vi "MyTestVI.vi"() -> ()   [LabVIEW 2018]
panel:
  in  "Stop Button":bool
  in  "test":bool
  out "error out":errorcluster
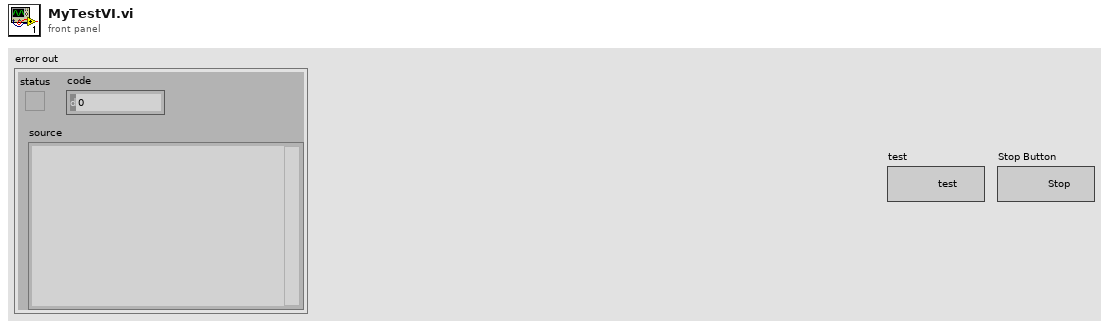
[diagram p1: front panel]
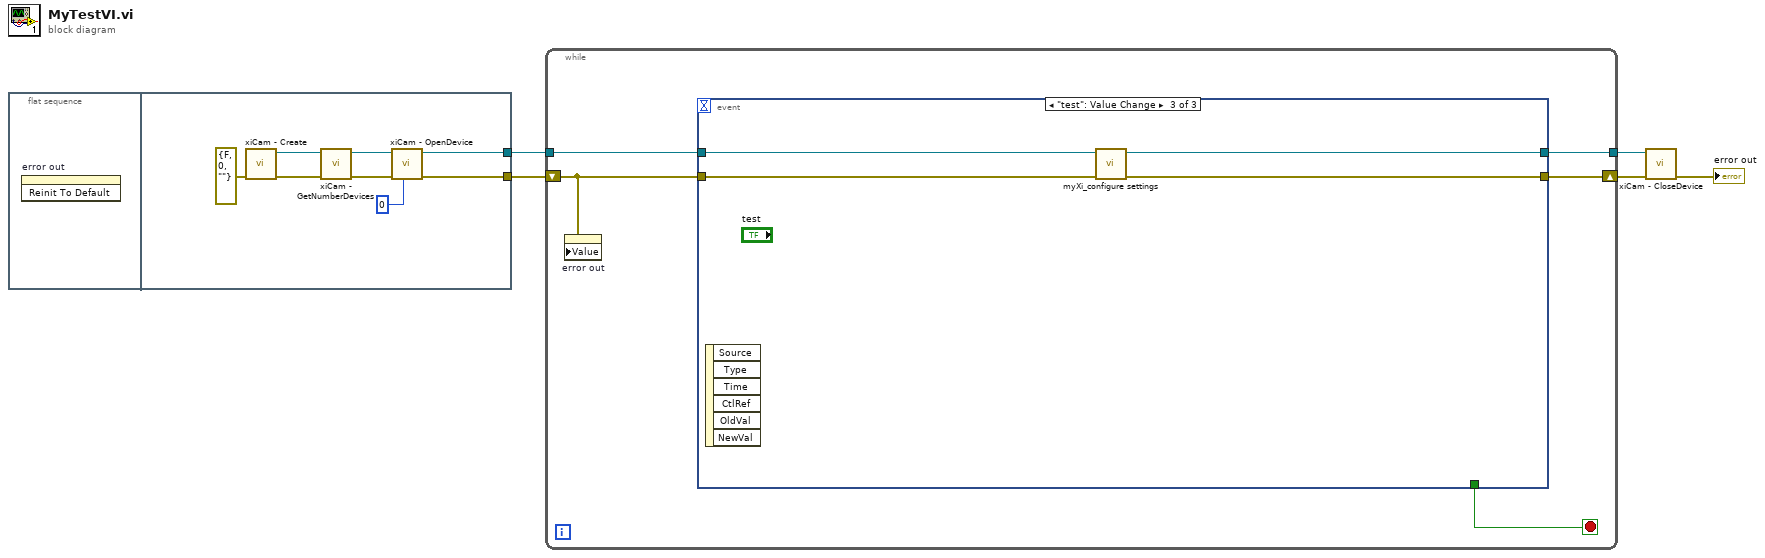
[diagram p0: block diagram]
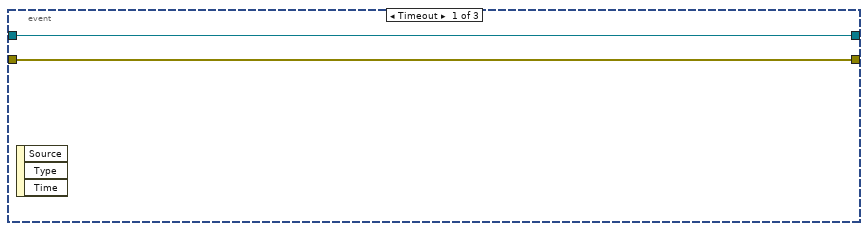
[diagram p2: hidden frame]
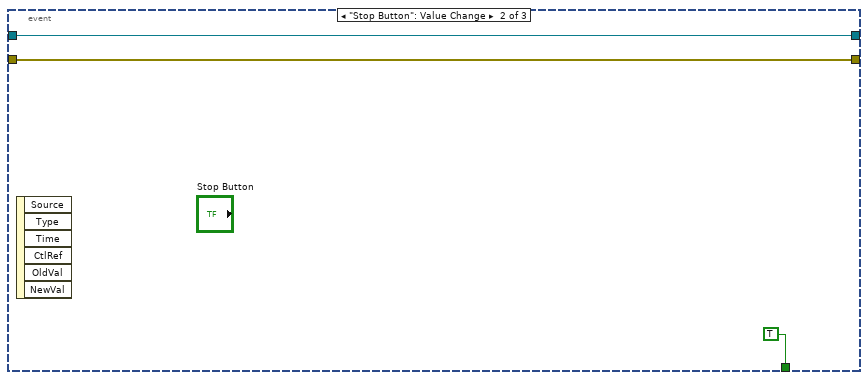
[diagram p3: hidden frame]
diagram:
  n1 = flat-sequence {
    tunnel: [w7] -> w3
    tunnel: [w6] -> w2
    frame #0 {
      n2 = invoke on="error out" class="Clust (strict)" method="Reinit To Default"() -> ()  [unwired: 3 in, 3 out]
    }
    frame #1 {
      n3 = call "xiCam - Create.vi"("error in (no error)"=errorcluster {"status"=FALSE, "code"=0, "source"=""}) -> ("error out"=w11:errorcluster, "new xiCam"=w10:refnum<k24>)  [unwired: 9 in]
      n4 = call "xiCam - GetNumberDevices.vi"("error in (no error)"=w11, "xiCam In"=w10) -> ("error out"=w13:errorcluster, "xiCam Out"=w12:refnum<k24>)  [unwired: 7 in, 1 out]
      n5 = call "xiCam - OpenDevice.vi"("DevID"=0, "error in (no error)"=w13, "xiCam In"=w12) -> ("error out"=w6:errorcluster, "xiCam Out"=w7:refnum<k24>)  [unwired: 7 in]
    }
  }
  n6 = while {
    tunnel: w3 -> [w16]
    shift-right: [w15] -> w4
    shift-left: w2 -> [w17]
    tunnel: [w14] -> w1
    stop <- w18 stop-if-true
    n7 = property on="error out" class="Clust (strict)"("Value"=w17) -> ()  [unwired: 2 in, 2 out]
    n8 = event shown="[2] \"test\": Value Change" {
      selector: _ -> [_ _ _]
      dyn-events: _ -> [_ _ _]
      timeout: _ -> [_ _ _]
      tunnel: [_ TRUE _] -> w18
      tunnel: w17 -> [w19 w22 w26]
      tunnel: w16 -> [w20 w21 w27]
      tunnel: [w19 w22 w24] -> w15
      tunnel: [w20 w21 w25] -> w14
      event Timeout {
        n9 = event-data() -> ()  [unwired: 1 in, 3 out]
      }
      event "Stop Button": Value Change {
        n10 = event-data() -> ()  [unwired: 1 in, 6 out]
      }
      event "test": Value Change {
        n11 = event-data() -> ()  [unwired: 1 in, 6 out]
        n12 = call "myXi_configure settings.vi"("error IN"=w26, "xiCam In"=w27) -> ("error OUT"=w24:errorcluster, "xiCam Out"=w25:refnum<k24>)  [unwired: 8 in]
      }
    }
  }
  n13 = call "xiCam - CloseDevice.vi"("error in (no error)"=w4, "xiCam In"=w1) -> ("error out"=→"error out":errorcluster)  [unwired: 9 in]
